vi "Exit.vi"() -> ()   [LabVIEW 2012]
panel:
  out "Exit?":bool
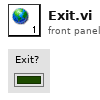
[diagram p1: front panel]
diagram:
